vi "Xsens RateOfTurn (SubVI).vi"(5 "DATA in (Hex)":string) -> (0 "Channel Units":string[](array[string])=["NA", "YYYY", "MM", "dd", "hh", "mm", "ss", "NA", "ns", "NA", "NA", "NA", "NA", "DD", "DD", "mm", "mm", "mm", "mm"], 1 "Channel DataTypes":string[](array[string])=["NA", "YYYY", "MM", "dd", "hh", "mm", "ss", "NA", "ns", "NA", "NA", "NA", "NA", "DD", "DD", "mm", "mm", "mm", "mm"], 2 "Rate of Turn":string[](array[string]), 3 "Channel Names":string[](array[string]))   [LabVIEW 2019]
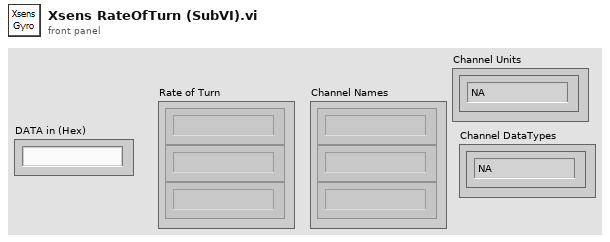
[diagram p1: front panel]
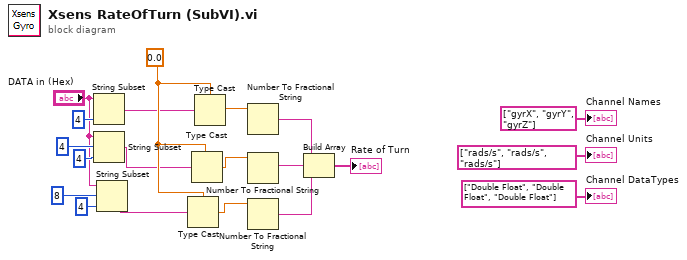
[diagram p0: block diagram]
diagram:
  w20 = sgl 0.0
  n1 = String Subset(string="DATA in (Hex)", length (rest)=4 ("length (rest)")) -> (substring=w18:string)  [unwired: 1 in]
  n2 = String Subset(string="DATA in (Hex)", offset (0)=4, length (rest)=4 ("length (rest)")) -> (substring=w13:string)
  n3 = String Subset(string="DATA in (Hex)", offset (0)=8, length (rest)=4 ("length (rest)")) -> (substring=w12:string)
  n4 = Type Cast(type=w20, x=w12) -> (*(type *) &x=w4:sgl)
  n5 = Type Cast(type=w20, x=w13) -> (*(type *) &x=w6:sgl)
  n6 = Type Cast(type=w20, x=w18) -> (*(type *) &x=w8:sgl)
  n7 = Number To Fractional String(number=w8) -> (F-format string=w7:string)  [unwired: 3 in]
  n8 = Number To Fractional String(number=w6) -> (F-format string=w5:string)  [unwired: 3 in]
  n9 = Number To Fractional String(number=w4) -> (F-format string=w3:string)  [unwired: 3 in]
  n10 = Build Array(w7, w5, w3) -> (→"Rate of Turn":string[])
  "Channel Names" <- string[] ["gyrX", "gyrY", "gyrZ"] ("Channel Names")
  "Channel Units" <- string[] ["rads/s", "rads/s", "rads/s"] ("Channel Names")
  "Channel DataTypes" <- string[] ["Double Float", "Double Float", "Double Float"] ("Channel Names")
